vi "GOMDBTS2048 calib Calculate Spectral Calibration Factors.vi"(8 "error in (no error)":errorcluster, 11 "handle":i32) -> (0 "error out":errorcluster, 2 "function return":i32, 3 "calFactors":dbl[](array[numeric]))   [LabVIEW 2015, in "GOMDBTS2048.lvlib"]
doc: "GOBTS2048DLL int __stdcall GOMDBTS2048_calibCalculateSpectralCalibrationFactors(int handle, double* calFactors);"
uses:
  GOMDBTS2048.lvlib
  runtime/GOMDBTS2048.dll
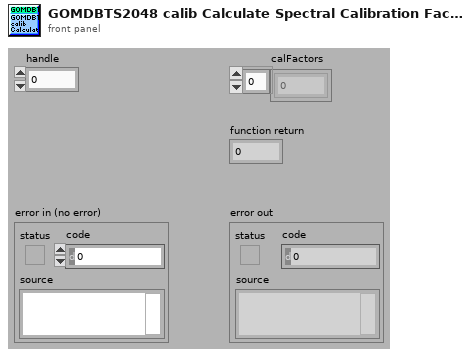
[diagram p1: front panel]
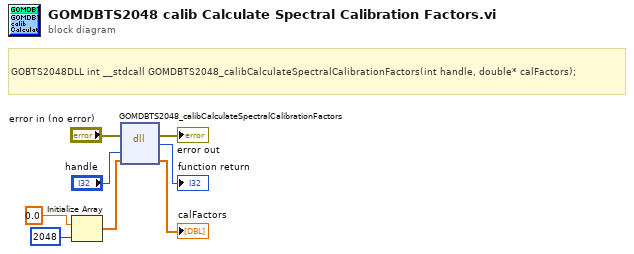
[diagram p0: block diagram]
diagram:
  # "GOBTS2048DLL int __stdcall GOMDBTS2048_calibCalculateSpectralCalibrationFactors(int handle, double* calFactors);"
  n1 = Initialize Array(0.0 ("element"), 2048 ("dimension size")) -> (w6:dbl[])
  n2 = dll-call lib="C:/Users/rkoch/Documents/GO_Library/runtime/GOMDBTS2048.*" fn="GOMDBTS2048_calibCalculateSpectralCalibrationFactors"(error in="error in (no error)", "handle"="handle", "calFactors"=w6) -> (error out=→"error out":errorcluster, →"function return":i32, "calFactors"=→"calFactors":dbl[])  [unwired: 3 in, 1 out]
